vi "log motor epics.vi"(6 "status":bool, 7 "Param Cluster":T1, 8 "Info":string, 9 "Position":dbl format="%#.6g", 10 "Command":string, 11 "IOC":string) -> (2 "Motor TextLog":string, 3 "Motor Log":string[][](array[string])=[["IOC"], ["Command"], ["Status"], ["Position"], ["Info"]])   [LabVIEW 2022 SP3]
uses:
  pectus/control/Param Epics Cluster.ctl
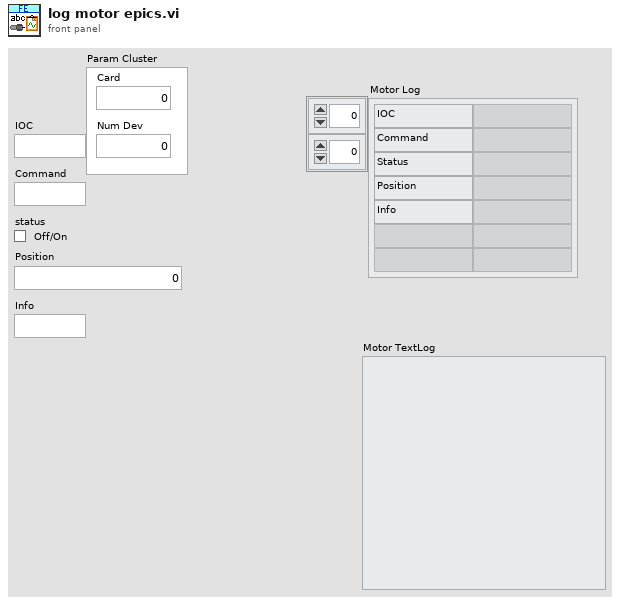
[diagram p1: front panel]
types:
  T1 = typedef "Param Epics Cluster.ctl" = cluster{"Card":u16, "Num Dev":u16}
  T2 = typedef "ca cluster.ctl" = cluster{"record":string, "prefix":string, "CA":string}
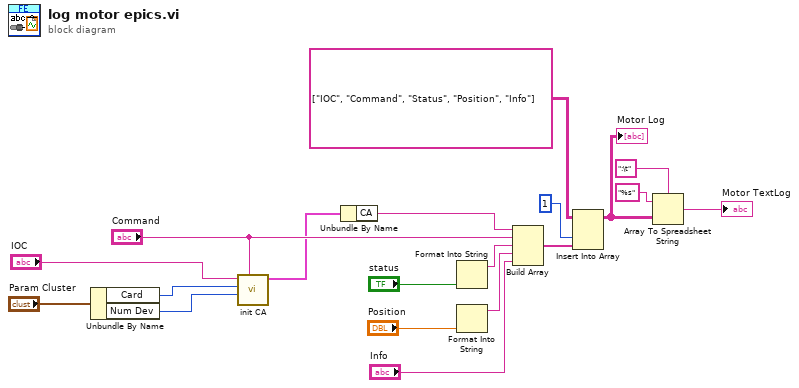
[diagram p0: block diagram]
diagram:
  n1 = Unbundle By Name("Param Cluster") -> ("Card"=w5:u16, "Num Dev"=w4:u16)
  n2 = call "init CA.vi"("Command"="Command", "Device"=w4, "Card"=w5, "IOC"="IOC") -> ("CA out"=w2:T2)  [unwired: 6 in, 1 out]
  n3 = Unbundle By Name(w2) -> ("CA"=w1:string)
  n4 = Format Into String("status") -> (resulting string=w15:string)  [unwired: 3 in, 1 out]
  n5 = Format Into String("Position") -> (resulting string=w17:string)  [unwired: 3 in, 1 out]
  n6 = Build Array(w1, "Command", w15, w17, "Info") -> (w13:string[])
  n7 = Insert Into Array(array=string[][] [["IOC"], ["Command"], ["Status"], ["Position"], ["Info"]], index (col)=1 ("disabled index (col)"), new element=w13) -> (w11:string[][])  [unwired: 1 in]
  "Motor Log" <- w11
  n8 = Array To Spreadsheet String(delimiter (Tab)=":\t", array=w11, 3:"%s" ("format string")) -> (spreadsheet string=→"Motor TextLog":string)
